vi "Version 1_Peak Detector.vi"(1 "Last Peak":dbl, 2 "New Value":dbl) -> (0 "Current Peak":dbl)   [LabVIEW 2015]
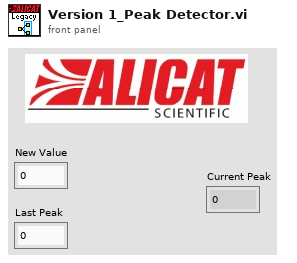
[diagram p1: front panel]
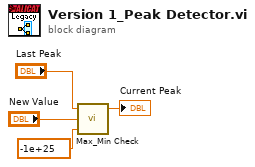
[diagram p0: block diagram]
diagram:
  n1 = call "Max_Min Check.vi"("Last Minimum"=-1e+25, "New Value"="New Value", "Last Maximum"="Last Peak") -> ("Maximum"=→"Current Peak":dbl)  [unwired: 1 in, 1 out]
